vi "call dll pointer.vi"() -> ()   [LabVIEW 2020]
uses:
  GPS_SIM_CREATE_BIN.dll
panel:
  out "output":i16[](array[numeric])
  out "error out":errorcluster
  in  "base_path":string="C:\\Users\\duyga\\OneDrive\\デスクトップ\\WORKS\\Nissan GPS\\build dll"
  in  "param":string="-e brdc0010.22n -l 36.318462,138.996902,0 -o gps_file -s 1000000 -b 16 -T 2023/06/28,18:39:03.511"
  out "res":i64
  # "iq8_buff[isamp] = iq_buff[isamp]>>4;"
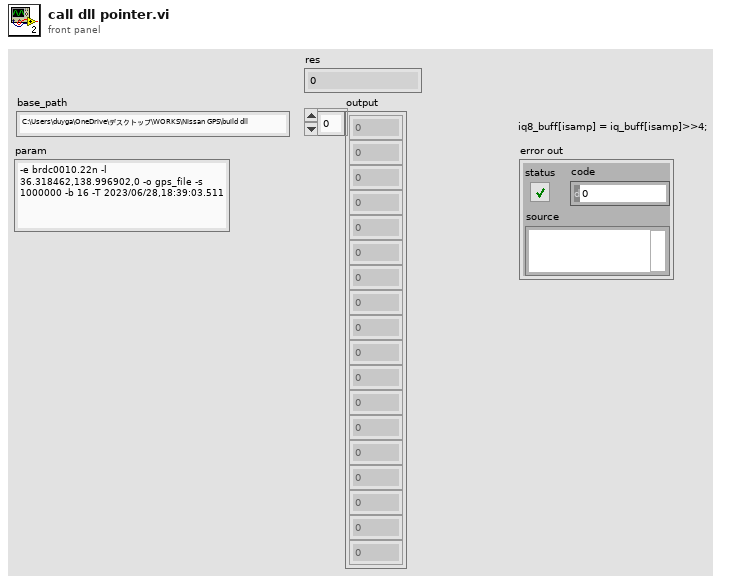
[diagram p1: front panel]
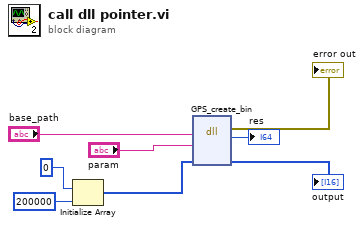
[diagram p0: block diagram]
diagram:
  n1 = Initialize Array(i16 0 ("element"), 200000 ("dimension size")) -> (w1:i16[])
  n2 = dll-call lib="PTH2iabs CUsersduygaOneDriveデスクトップWORKS\nNissan GPS\tbuild dllGPS_SIM_CREATE_BIN.dll" fn="GPS_create_bin"("param"="param", "base_path"="base_path", "output"=w1) -> (error out=→"error out":errorcluster, "IQ data"=→"res":i64, "output"=→"output":i16[])  [unwired: 5 in, 1 out]
